vi "getNumChannels.vi"(8 "error in (no error)":errorcluster, 11 "DAQ in":refnum<class "DAQ.lvclass">) -> (0 "error out":errorcluster, 2 "NumChannels":i32, 3 "DAQ out":refnum<class "DAQ.lvclass">)   [LabVIEW 2016, in "DAQ.lvclass"]
uses:
  DAQ.lvclass
  DAQ.lvclass/DAQ.ctl
  <vilib>/regexp/Match Regular Expression.xnode
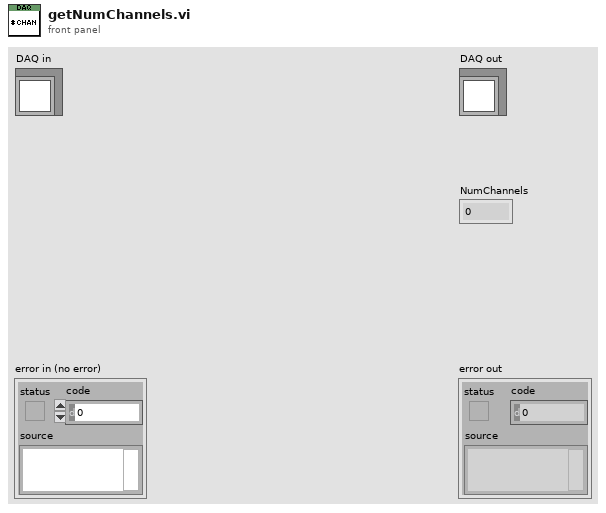
[diagram p1: front panel]
types:
  T1 = typedef "DAQ.lvclass/PrivateEvents--DAQ.AI.Channels.ctl" = string
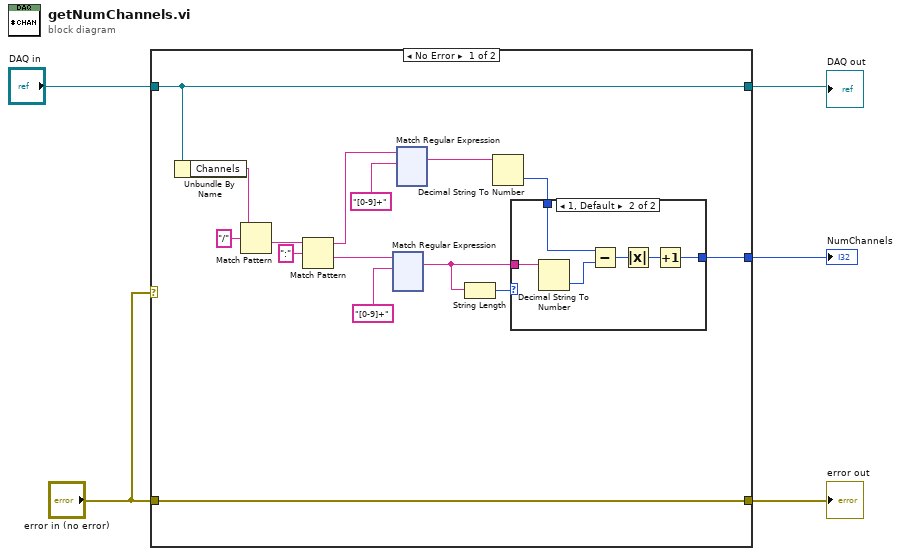
[diagram p0: block diagram]
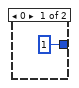
[diagram p2: hidden frame]
diagram:
  n1 = case shown="No Error" "error in (no error)" {
    tunnel: [w20 _] -> w5
    tunnel: "DAQ in" -> [w7 w256]
    tunnel: "error in (no error)" -> [w6 w257]
    tunnel: [w7 w256] -> w2
    tunnel: [w6 w257] -> w1
    frame No Error {
      n2 = Unbundle By Name(w7) -> ("Channels"=w8:T1)
      n3 = Match Pattern(string=w8, regular expression="/") -> (after substring=w11:T1)  [unwired: 1 in, 3 out]
      n4 = Match Pattern(string=w11, regular expression=":") -> (before substring=w16:T1, after substring=w15:T1)  [unwired: 1 in, 2 out]
      n5 = xnode "Match Regular Expression"("input string"=w15, "regular expression"="[0-9]+") -> ("whole match"=w18:string)  [unwired: 4 in, 4 out]
      n6 = xnode "Match Regular Expression"("input string"=w16, "regular expression"="[0-9]+") -> ("whole match"=w13:string)  [unwired: 4 in, 4 out]
      n7 = String Length(string=w18) -> (length=w19:i32)
      n8 = Decimal String To Number(string=w13) -> (number=w14:i32)  [unwired: 2 in, 1 out]
      n9 = case shown="1, Default" w19 {
        tunnel: w14 -> [_ w27]
        tunnel: [1 w23] -> w20
        tunnel: w18 -> [_ w22]
        frame 0 {
        }
        frame 1, Default {
          n10 = Decimal String To Number(string=w22) -> (number=w26:i32)  [unwired: 2 in, 1 out]
          n11 = Subtract(x=w27, y=w26) -> (x-y=w25:i32)
          n12 = Absolute Value(x=w25) -> (abs(x)=w24:i32)
          n13 = Increment(x=w24) -> (x+1=w23:i32)
        }
      }
    }
    frame Error {
    }
  }
  "NumChannels" <- w5
  "error out" <- w1
  "DAQ out" <- w2
